vi "Configuration parameter reading.vi"(8 "error in (no error)":errorcluster caption="错误输入（无错误）") -> (0 "error out":errorcluster caption="错误输出", 1 "enable":bool, 2 "baud rate (9600)":u32(ring)=4800 caption="波特率" items=["1200"=1200, "2400"=2400, "4800"=4800, "9600"=9600, "19200"=19200, "38400"=38400, "115200"=115200], 3 "VISA resource name":refnum<visa-resource-name> caption="串口", 4 "Shift distance":u32)   [LabVIEW 2016, in "环境动力监测库.lvlib" / "AIRMAR WeatherCaster.lvlib"]
uses:
  AIRMAR WeatherCaster.lvlib
  <vilib>/Utility/config.llb/Read Key (String).vi
  <vilib>/Utility/config.llb/Read Key (U32).vi
  <vilib>/Utility/config.llb/Read Key (Boolean).vi
  <vilib>/Utility/config.llb/NI_LVConfig.lvlib
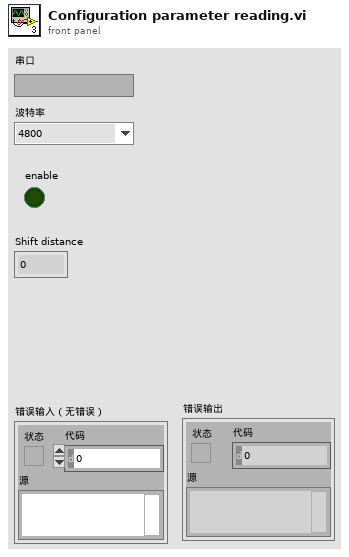
[diagram p1: front panel]
types:
  T1 = cluster{"监测项描述:输出":string, "连接方式":enum16{"串口", "TCP"}, "端口":string, "IP address:":string, "Port:":string, "站号":u64, "传感器型号":string, "波特率":u64, "data bits":u64, "停止位":u16, "奇偶校验":u16}
  T2 = typedef "NI_LVConfig.lvlib/Config Data RefNum.ctl" = refnum<k1>
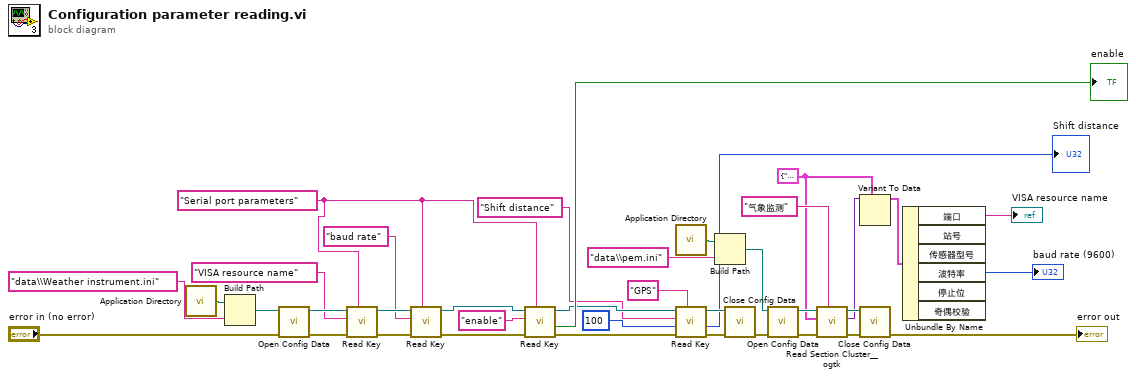
[diagram p0: block diagram]
diagram:
  w5 = T1 {"监测项描述:输出"="", "连接方式"=enum."串口", "端口"="", "IP address:"="", "Port:"="", "站号"=19200, "传感器型号"="", "波特率"=19200, "data bits"=8, "停止位"=10, "奇偶校验"=0} ("输入簇")
  w26 = "Serial port parameters" ("section")
  n1 = call <vilib>:"Application Directory.vi"() -> ("Application Directory"=w35:path)
  n2 = Build Path(base path=w35, name or relative path="data\\Weather instrument.ini" ("名称或相对路径")) -> (appended path=w36:path)
  n3 = call <vilib>:"Open Config Data.vi"("error in (no error)"="error in (no error)", "configuration file path"=w36) -> ("error out"=w37:errorcluster, "refnum"=w38:T2)  [unwired: 7 in, 1 out]
  n4 = call-poly <vilib>:"Read Key.vi"("section"=w26, "error in (no error)"=w37, "key"="VISA resource name", "refnum"=w38) -> ("error out"=w31:errorcluster, "refnum out"=w32:T2)  [unwired: 4 in, 2 out]
  n5 = call-poly <vilib>:"Read Key.vi"("section"=w26, "error in (no error)"=w31, "key"="baud rate", "refnum"=w32) -> ("error out"=w27:errorcluster, "refnum out"=w28:T2)  [unwired: 4 in, 2 out]
  n6 = call-poly <vilib>:"Read Key.vi"("section"=w26, "error in (no error)"=w27, "key"="enable", "refnum"=w28) -> ("error out"=w21:errorcluster, "value"=→"enable":bool, "refnum out"=w23:T2)  [unwired: 4 in, 1 out]
  n7 = call <vilib>:"Application Directory.vi"() -> ("Application Directory"=w12:path)
  n8 = call-poly <vilib>:"Read Key.vi"("section"="GPS", "error in (no error)"=w21, "default value"=u32 100, "key"="Shift distance" ("section"), "refnum"=w23) -> ("error out"=w20:errorcluster, "value"=→"Shift distance":u32, "refnum out"=w22:T2)  [unwired: 3 in, 1 out]
  n9 = Build Path(base path=w12, name or relative path="data\\pem.ini" ("名称或相对路径")) -> (appended path=w13:path)
  n10 = call <vilib>:"Close Config Data.vi"("error in (no error)"=w20, "refnum"=w22) -> ("error out"=w4:errorcluster)  [unwired: 8 in, 1 out]
  n11 = call <vilib>:"Open Config Data.vi"("error in (no error)"=w4, "configuration file path"=w13) -> ("error out"=w14:errorcluster, "refnum"=w15:T2)  [unwired: 7 in, 1 out]
  n12 = call <userlib>:"Read Section Cluster__ogtk.vi"("section (optional)"="气象监测", "error in (no error)"=w14, "Section Formatted Cluster Type"=w5, "refnum"=w15) -> ("error out"=w8:errorcluster, "Section Formatted Cluster"=w7:variant, "dup refnum"=w9:T2)  [unwired: 3 in, 2 out]
  n13 = Variant To Data(type=w5, Variant=w7) -> (data=w6:T1)  [unwired: 1 in, 1 out]
  n14 = call <vilib>:"Close Config Data.vi"("error in (no error)"=w8, "refnum"=w9) -> ("error out"=→"error out":errorcluster)  [unwired: 8 in, 1 out]
  n15 = Unbundle By Name(w6) -> ("端口"=→"VISA resource name":string, "波特率"=→"baud rate (9600)":u64)  [unwired: 4 out]
